vi "Stop.vi"(8 "error in (no error)":errorcluster, 10 "Message in":refnum<class "StopMessage.lvclass">, 11 "Autofocus in":refnum<class "Autofocus.lvclass">) -> (0 "error out":errorcluster, 3 "Autofocus out":refnum<class "Autofocus.lvclass">)   [LabVIEW 2012, in "Autofocus.lvclass"]
doc: "This member function is called when the statemachine in the run.vi receives an 'stop' command. It relays the message to all observers of the component.\n\nOverride this member function in your derived class if you need additional stop functionality (but don't forget to call the parent method)."
uses:
  Autofocus.lvclass
  <vilib>/Distrio/Murmex/StopMessage/StopMessage.lvclass
  <vilib>/Distrio/Murmex/Murmex/Murmex.lvclass
  Autofocus.lvclass/Autofocus.ctl
  <vilib>/Utility/file.llb/Write To Spreadsheet File (DBL).vi
panel:
  out "stack duration":dbl
  # "This method is called when the STOP\ntrigger is sent. \n\nOverride this method when your component needs to\nrespond to this trigger. \n\nCall parent for proper implementation"
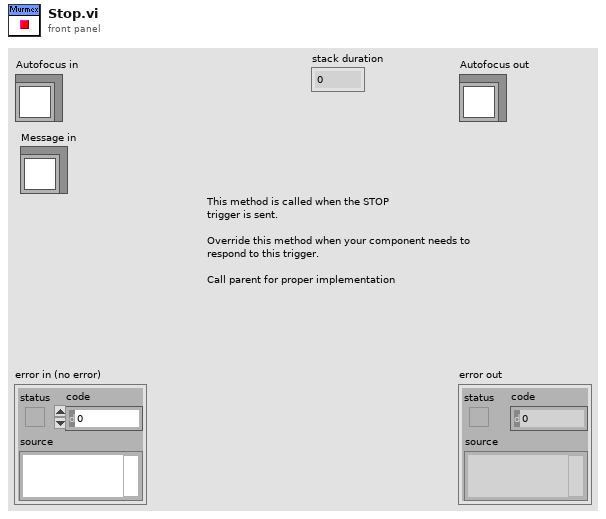
[diagram p1: front panel]
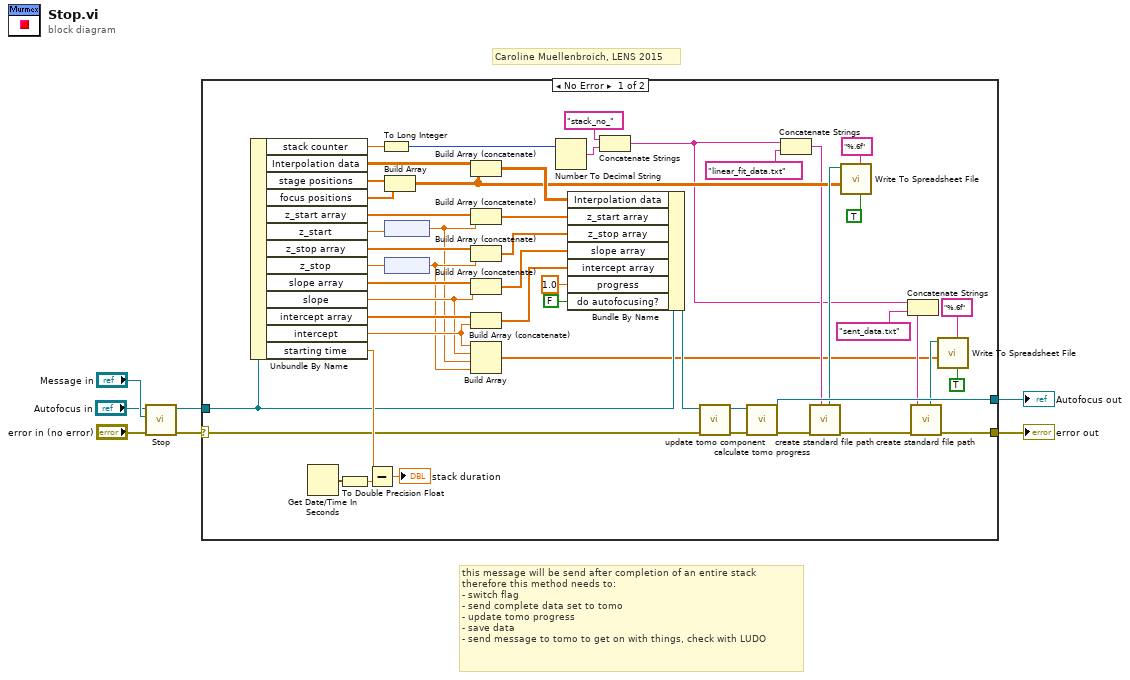
[diagram p0: block diagram]
diagram:
  # "Caroline Muellenbroich, LENS 2015"
  # "this message will be send after completion of an entire stack\ntherefore this method needs to:\n- switch flag\n- send complete data set to tomo\n- update tomo progress\n- save data\n- send message to tomo to get on with things, check with LUDO"
  n1 = call-parent "Stop.vi"("error in (no error)"="error in (no error)", "Message in"="Message in", "Murmex in"="Autofocus in") -> ("error out"=w4:errorcluster, "Murmex out"=w3:refnum<class "Autofocus.lvclass">)  [unwired: 7 in]
  n2 = case shown="No Error" w4 {
    selector: w4 -> [w52 w59]
    tunnel: w3 -> [w31 w58]
    tunnel: [w21 w59] -> w2
    tunnel: [w49 w58] -> w1
    frame No Error {
      n3 = Unbundle By Name(w31) -> ("stack counter"=w32:dbl, "Interpolation data"=w27:dbl[][][], "stage positions"=w26:dbl[], "focus positions"=w25:dbl[], "z_start array"=w29:dbl[], "z_start"=w30:dbl[unit], "z_stop array"=w34:dbl[], "z_stop"=w35:dbl[unit], "slope array"=w37:dbl[], "slope"=w11:dbl, "intercept array"=w39:dbl[], "intercept"=w12:dbl, "starting time"=w56:dbl)
      n4 = Get Date/Time In Seconds() -> (seconds since 1Jan1904=w57:timestamp)
      n5 = To Double Precision Float(number=w57) -> (double precision float=w55:dbl)
      n6 = Subtract(x=w56, y=w55) -> (x-y=→"stack duration":dbl)
      n7 = To Long Integer(number=w32) -> (32bit integer=w46:i32)
      n8 = Build Array(w26, w25) -> (w23:dbl[][])
      n9 = node(w30) -> (w9:dbl)
      n10 = node(w35) -> (w10:dbl)
      n11 = Build Array (concatenate)(w27, w23) -> (w24:dbl[][][])
      n12 = Build Array (concatenate)(w29, w9) -> (w28:dbl[])
      n13 = Build Array (concatenate)(w34, w10) -> (w33:dbl[])
      n14 = Build Array (concatenate)(w37, w11) -> (w36:dbl[])
      n15 = Build Array (concatenate)(w39, w12) -> (w38:dbl[])
      n16 = Build Array(w12, w11, w9, w10) -> (w8:dbl[])
      n17 = Number To Decimal String(number=w46) -> (decimal integer string=w45:string)  [unwired: 1 in]
      n18 = Bundle By Name(cluster=w31, "Interpolation data"=w24, "z_start array"=w28, "z_stop array"=w33, "slope array"=w36, "intercept array"=w38, "progress"=1.0 ("Runtime cluster.Stack.progress"), "do autofocusing?"=FALSE ("Runtime cluster.Stack.do autofocusing?")) -> (w51:refnum<class "Autofocus.lvclass">)
      n19 = Concatenate Strings("stack_no_" ("string"), w45) -> (w13:string)
      n20 = call-dynamic "update tomo component.vi"("error in (no error)"=w52, "Autofocus in"=w51) -> ("error out"=w48:errorcluster, "Autofocus out"=w50:refnum<class "Autofocus.lvclass">)  [unwired: 8 in]
      n21 = call-dynamic "calculate tomo progress.vi"("error in (no error)"=w48, "Autofocus in"=w50) -> ("error out"=w43:errorcluster, "Autofocus out"=w49:refnum<class "Autofocus.lvclass">)  [unwired: 8 in]
      n22 = Concatenate Strings(w13, "linear_fit_data.txt" ("string")) -> (w16:string)
      n23 = call "create standard file path.vi"("name or relative path"=w16, "error in (no error)"=w43) -> ("error out"=w22:errorcluster, "appended path"=w40:path)  [unwired: 8 in]
      n24 = call-poly <vilib>:"Write To Spreadsheet File.vi"("transpose? (no:F)"=TRUE, "format (%.3f)"="%.6f", "2D data"=w23, "file path (dialog if empty)"=w40) -> ()  [unwired: 2 in, 3 out]
      n25 = Concatenate Strings(w13, "sent_data.txt" ("string")) -> (w14:string)
      n26 = call "create standard file path.vi"("name or relative path"=w14, "error in (no error)"=w22) -> ("error out"=w21:errorcluster, "appended path"=w19:path)  [unwired: 8 in]
      n27 = call-poly <vilib>:"Write To Spreadsheet File.vi"("transpose? (no:F)"=TRUE, "format (%.3f)"="%.6f", "1D data"=w8, "file path (dialog if empty)"=w19) -> ()  [unwired: 2 in, 3 out]
    }
    frame Error {
    }
  }
  "error out" <- w2
  "Autofocus out" <- w1
